vi "Set FC1.vi"(10 "FC1":refnum<class "Actuator Cylinder.lvclass">, 11 "SingleCylinderActuator in":refnum<class "Dual Cylinder Outer Loop Actuator.lvclass">) -> (3 "SingleCylinderActuator out":refnum<class "Dual Cylinder Outer Loop Actuator.lvclass">)   [LabVIEW 2015, in "Dual Cylinder Outer Loop Actuator.lvclass"]
uses:
  Dual Cylinder Outer Loop Actuator.lvclass
  Actuator Cylinder/Actuator Cylinder/Actuator Cylinder.lvclass
  Dual Cylinder Outer Loop Actuator.lvclass/Dual Cylinder Outer Loop Actuator.ctl
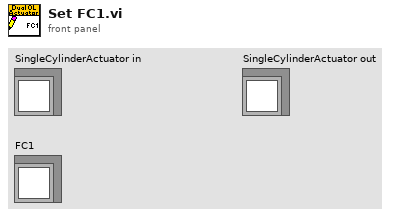
[diagram p1: front panel]
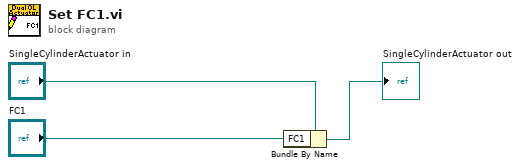
[diagram p0: block diagram]
diagram:
  n1 = Bundle By Name(cluster="SingleCylinderActuator in", "FC1"="FC1") -> (→"SingleCylinderActuator out":refnum<class "Dual Cylinder Outer Loop Actuator.lvclass">)
